vi "ReadPower.vi"(8 "error in":errorcluster, 11 "TE Cooler in":refnum<class "TE Cooler.lvclass">) -> (0 "error out":errorcluster, 2 "Power (%)":sgl, 3 "TE Cooler out":refnum<class "TE Cooler.lvclass">)   [LabVIEW 2018, in "TE Cooler.lvlib" / "TE Cooler.lvclass"]
doc: "Read the power being used currently by the controller (-100 to 100%). Uses the command <B>POWER OUTPUT</ B>."
uses:
  TE Cooler.lvclass
  Controls/Command.ctl
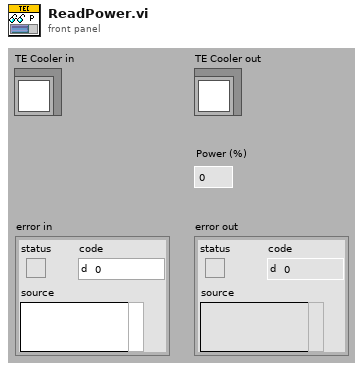
[diagram p1: front panel]
types:
  T1 = typedef "TE Cooler.lvlib/TE Cooler.lvclass/Command.ctl" = enum16{"INPUT1", "DESIRED CONTROL VALUE", "POWER OUTPUT", "ALARM STATUS", "INPUT 2", "OUTPUT CURRENT COUNTS", "ALARM TYPE", "SET TYPE DEFINE", "SENSOR TYPE", "CONTROL TYPE", "CONTROL OUTPUT POLARITY", "POWER ON/OFF", "OUTPUT SHUTDOWN IF ALARM", "FIXED DESIRED CONTROL SETTING", "PROPORTIONAL BANDWIDTH", "INTEGRAL GAIN", "DERIVATIVE GAIN", "LOW EXTERNAL SET RANGE", "HIGH EXTERNAL SET RANGE", "ALARM DEADBAND", "HIGH ALARM SETTING", "LOW ALARM SETTING", "CONTROL DEADBAND SETTING", "INPUT1 OFFSET", "INPUT2 OFFSET", "HEAT MULTIPLIER", "COOL MULTIPLIER", "OVER CURRENT COUNT COMPARE VALUE", "ALARM LATCH ENABLE", "NOT USED", "ALARM LATCH RESET", "CHOOSE SENSOR FOR ALARM FUNCTION", "CHOOSE TEMPERATURE WORKING UNITS", "EEPROM WRITE ENABLE", "OVER CURRENT CONTINUOUS", "OVER CURRENT RESTART ATTEMPTS", "JP3 DISPLAY ENABLE"}
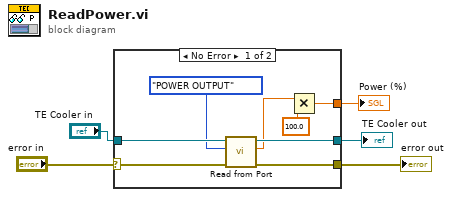
[diagram p0: block diagram]
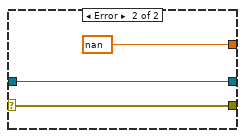
[diagram p2: hidden frame]
diagram:
  n1 = case shown="No Error" "error in" {
    selector: "error in" -> [w13 w16]
    tunnel: [w11 w16] -> w3
    tunnel: "TE Cooler in" -> [w12 w15]
    tunnel: [w10 w15] -> w4
    tunnel: [w6 sgl nan ("scaledOut")] -> w1
    frame No Error {
      n2 = call "Read from Port.vi"("error in"=w13, "TEC Cmd"=Command."POWER OUTPUT", "TE Cooler in"=w12) -> ("error out"=w11:errorcluster, "scaledOut"=w8:sgl, "TE Cooler out"=w10:refnum<class "TE Cooler.lvclass">)  [unwired: 5 in, 1 out]
      n3 = Multiply(x=w8, y=sgl 100.0) -> (x*y=w6:sgl)
    }
    frame Error {
    }
  }
  "error out" <- w3
  "TE Cooler out" <- w4
  "Power (%)" <- w1
